vi "RT.vi"() -> ()   [LabVIEW 2015]
uses:
  <vilib>/FPGAPlugInAG/sbRIO-9637/niLvFpga_Open_sbRIO-9637.vi
  <vilib>/rvi/interface/common/dynamic/niFpgaDynamicAddResources.vi
  <vilib>/Utility/error.llb/Error Cluster From Error Code.vi
  <vilib>/rvi/errors/niLvFpgaAdjustHostInterfaceError.vi
  <vilib>/FPGAPlugInAG/Dynamic/niLvFpga_Close_Dynamic.vi
  <vilib>/EmbeddedDisplay/Hitachi HD44780/Host/Public/Output (String).vi
  <vilib>/rvi/interface/nirviOpenFPGA/nirviOpenFPGA.xnode
  FPGA Bitfiles/ECM-Project_FPGATarget_FPGA_qZxlCAm-DOY.lvbitx
  FPGA/FPGA.vi
  <vilib>/rvi/interface/nirviReadWriteControl/nirviReadWriteControl.xnode
  <vilib>/rvi/interface/nirviCloseFPGA/nirviCloseFPGA.xnode
  <vilib>/rvi/interface/nirviMethod/nirviMethod.xnode
  <vilib>/EmbeddedDisplay/Hitachi HD44780/Host/HD44780 Host.lvlib
  <vilib>/FPGAPlugInAG/Dynamic/niLvFpga_ReadFifo_Dynamic.vi
  <vilib>/rvi/errors/niLvFpgaMergeErrorWithErrorCode.vi
  NiFpgaLv.dll
  <vilib>/rvi/interface/Simulation/niFpgaSimulationCallBeginRW.vi
panel:
  out "Gauge":dbl(knob) scale=0.0..10.0
  out "Meter":dbl(knob) scale=0.0..5.0
  in  "Port":u16=2055 min=1025 step=1
  in  "Clear LCD":bool
  in  "Slide":dbl(slide) scale=0.0..10.0
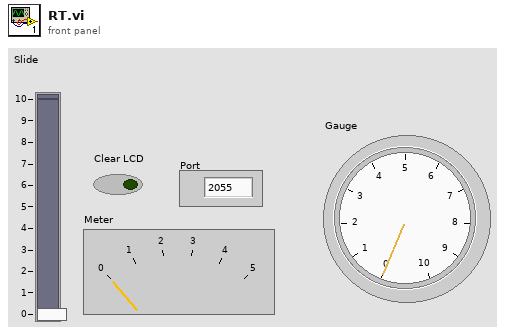
[diagram p1: front panel]
types:
  T1 = enum8{"5x8 & 2 lines", "5x10 & 1 line", "5x8 & 1 line"}
  T2 = enum8{"8x1", "8x2", "12x4", "16x1", "16x2", "16x4", "20x1", "20x2", "20x4", "24x1", "24x2", "40x2", "40x4"}
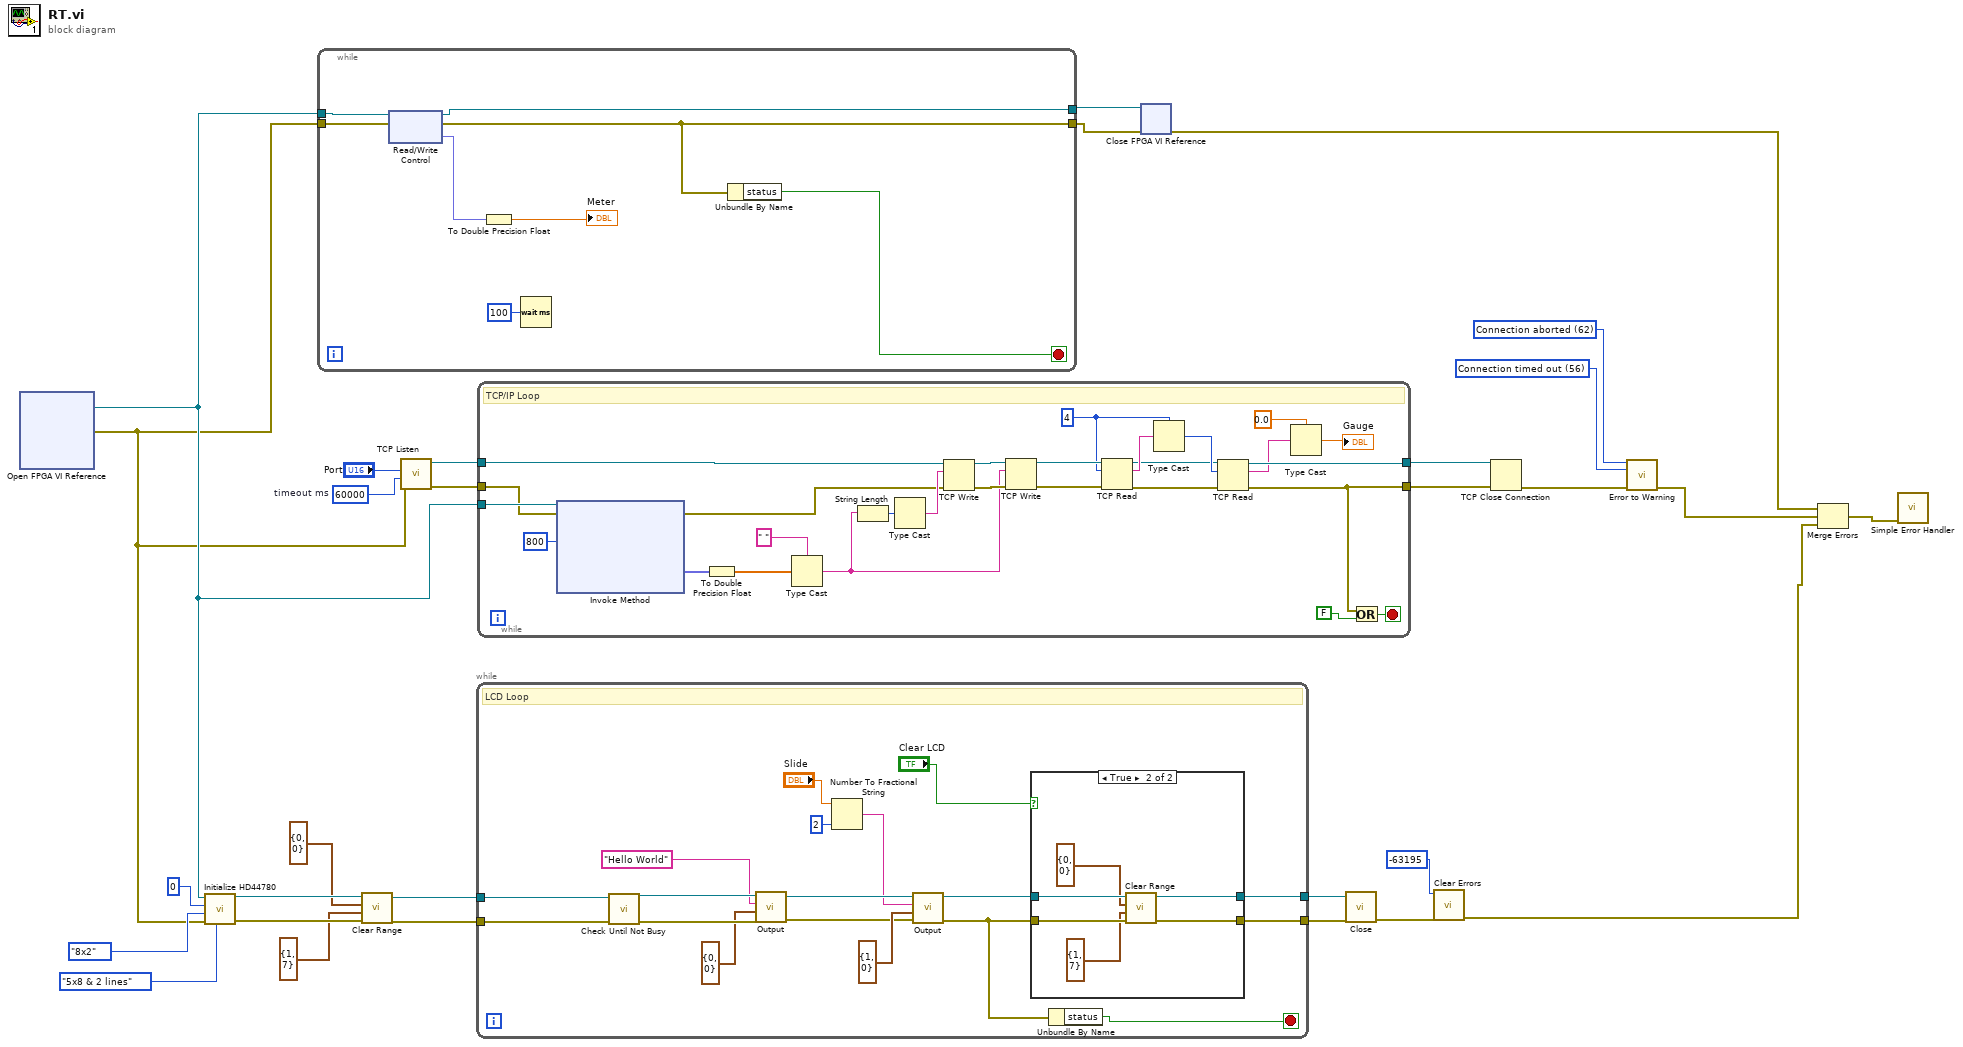
[diagram p0: block diagram]
diagram:
  w17 = 60000  # timeout ms
  w12 = 56 items=["No Error", "Argument Error", "Memory Full", "Out of Zone", "End of File", "File Already Open", "Generic File IO Error", "File Not Found", "File Permission Error", "Disk Full", "Duplicate Path", "Too Many Files Open", "Not Enabled", "Resource File Not Found", "Cannot Add Resource", "Resource Not Found", "Image Not Found", "Image Memory Error", "Pen Does Not Exist", "Config Bad Type", "Config Token Not Found", "Config Parse Error", "Config Memory Error", "Bad External Code Format", "Bad External Code Offset", "External Code Not Present", "Null Window", "Destroy Window Mixup", "Null Menu", "Print Aborted", "Bad Print Record", "Print Driver Error", "Windows Error During Print", "Memory Error During Print", "Print Dialog Error", "Generic Print Error", "Invalid Device Refnum", "Device Not Found", "Device Parameter Error", "Device Unit Error", "Can't Open Device", "Device Call Aborted", "Generic Error", "Cancelled By User", "Object ID Too Low", "Object ID Too High", "Object Not In Heap", "Unknown Heap", "Bad DefProc ID", "DefProc Not In Table", "Message Out Of Range", "Null Method", "Unknown Message", "Manager Call Not Supported", "Bad address", "Connection In progress", "Connection timed out", "Connection is already in progress", "Network attribute not supported", "Network error", "Address in use", "System out of memory", "Connection aborted", "Connection refused", "Connection is not connected", "Connection is already connected", "Connection closed", "Initialize error (interapplication manager)", "Bad occurrence", "Wait on unbound occurrence handler", "Occurrence queue overflow", "Bad path", "Semaphore not signaled", "Unrecognized type (interapplication manager)"] ("2nd Error to Convert")
  w11 = 62 items=["No Error", "Argument Error", "Memory Full", "Out of Zone", "End of File", "File Already Open", "Generic File IO Error", "File Not Found", "File Permission Error", "Disk Full", "Duplicate Path", "Too Many Files Open", "Not Enabled", "Resource File Not Found", "Cannot Add Resource", "Resource Not Found", "Image Not Found", "Image Memory Error", "Pen Does Not Exist", "Config Bad Type", "Config Token Not Found", "Config Parse Error", "Config Memory Error", "Bad External Code Format", "Bad External Code Offset", "External Code Not Present", "Null Window", "Destroy Window Mixup", "Null Menu", "Print Aborted", "Bad Print Record", "Print Driver Error", "Windows Error During Print", "Memory Error During Print", "Print Dialog Error", "Generic Print Error", "Invalid Device Refnum", "Device Not Found", "Device Parameter Error", "Device Unit Error", "Can't Open Device", "Device Call Aborted", "Generic Error", "Cancelled By User", "Object ID Too Low", "Object ID Too High", "Object Not In Heap", "Unknown Heap", "Bad DefProc ID", "DefProc Not In Table", "Message Out Of Range", "Null Method", "Unknown Message", "Manager Call Not Supported", "Bad address", "Connection In progress", "Connection timed out", "Connection is already in progress", "Network attribute not supported", "Network error", "Address in use", "System out of memory", "Connection aborted", "Connection refused", "Connection is not connected", "Connection is already connected", "Connection closed", "Initialize error (interapplication manager)", "Bad occurrence", "Wait on unbound occurrence handler", "Occurrence queue overflow", "Bad path", "Semaphore not signaled", "Unrecognized type (interapplication manager)"] ("1st Error to Convert")
  n1 = xnode "Open FPGA VI Reference"() -> ("FPGA VI Reference Out"=w5:refnum<k20>, "error out"=w4:errorcluster)  [unwired: 2 in]
  n2 = call <vilib>:"Initialize HD44780.vi"("font configuration (5x8 & 2 lines)"=T1."5x8 & 2 lines", "error in (no error)"=w4, "screen size"=T2."8x2", "device index"=i8 0, "FPGA VI Reference in"=w5) -> ("error out"=w21:errorcluster, "LCD out"=w20:refnum<class "Character LCD.lvclass">)  [unwired: 5 in]
  n3 = while {
    tunnel: w5 -> [w38]
    tunnel: w4 -> [w37]
    tunnel: [w33] -> w3
    tunnel: [w32] -> w2
    stop <- w34 stop-if-true
    n4 = xnode "Read/Write Control"("FPGA VI Reference In"=w38, "error in"=w37) -> ("FPGA VI Reference Out"=w33:refnum<k20>, "error out"=w32:errorcluster, "POT"=w36:fxp<+/-,24,5>)
    n5 = To Double Precision Float(number=w36) -> (double precision float=→"Meter":dbl)
    n6 = Wait (ms)(milliseconds to wait=u32 100) -> ()  [unwired: 1 out]
    n7 = Unbundle By Name(w32) -> ("status"=w34:bool)
  }
  n8 = call <vilib>:"Clear Range.vi"("error in (no error)"=w21, "end position (end of line)"=cluster{"row":i8, "column":i8} {"row"=1, "column"=7}, "start position"=cluster{"row":i8, "column":i8} {"row"=0, "column"=0}, "LCD in"=w20) -> ("error out"=w23:errorcluster, "LCD out"=w22:refnum<class "Character LCD.lvclass">)  [unwired: 6 in]
  n9 = call <vilib>:"TCP Listen.vi"("error in (no error)"=w4, "timeout ms (wait forever: -1)"=w17, "port"="Port") -> ("error out"=w16:errorcluster, "connection ID"=w14:refnum<k5>)  [unwired: 1 in, 6 out]
  n10 = while {
    tunnel: w22 -> [w55]
    tunnel: w23 -> [w56]
    tunnel: [w42] -> w25
    tunnel: [w41] -> w24
    stop <- w39 stop-if-true
    # "LCD Loop"
    n11 = call "Check Until Not Busy.vi"("error in"=w56, "LCD in"=w55) -> ("error out"=w54:errorcluster, "LCD out"=w53:refnum<class "Character LCD.lvclass">)  [unwired: 8 in]
    n12 = call-poly <vilib>:"Output.vi"("error in (no error)"=w54, "position"=cluster{"row":i8, "column":i8} {"row"=0, "column"=0}, "text"="Hello World" ("String"), "LCD in"=w53) -> ("error out"=w50:errorcluster, "LCD out"=w49:refnum<class "Character LCD.lvclass">)  [unwired: 5 in, 1 out]
    n13 = Number To Fractional String(number="Slide", precision (6)=i16 2) -> (F-format string=w46:string)  [unwired: 2 in]
    n14 = call-poly <vilib>:"Output.vi"("error in (no error)"=w50, "position"=cluster{"row":i8, "column":i8} {"row"=1, "column"=0}, "text"=w46, "LCD in"=w49) -> ("error out"=w40:errorcluster, "LCD out"=w43:refnum<class "Character LCD.lvclass">)  [unwired: 5 in, 1 out]
    n15 = case shown="True" "Clear LCD" {
      tunnel: w43 -> [w58 w64]
      tunnel: w40 -> [w57 w63]
      tunnel: [w57 w62] -> w42
      tunnel: [w58 w61] -> w41
      frame False {
      }
      frame True {
        n16 = call <vilib>:"Clear Range.vi"("error in (no error)"=w63, "end position (end of line)"=cluster{"row":i8, "column":i8} {"row"=1, "column"=7}, "start position"=cluster{"row":i8, "column":i8} {"row"=0, "column"=0}, "LCD in"=w64) -> ("error out"=w62:errorcluster, "LCD out"=w61:refnum<class "Character LCD.lvclass">)  [unwired: 6 in]
      }
    }
    n17 = Unbundle By Name(w40) -> ("status"=w39:bool)
  }
  n18 = while {
    tunnel: [w74] -> w15
    tunnel: [w73] -> w13
    tunnel: w14 -> [w91]
    tunnel: w16 -> [w82]
    tunnel: w5 -> [w83]
    stop <- w85 stop-if-true
    w70 = 4
    # "TCP/IP Loop"
    n19 = xnode "Invoke Method"("FPGA VI Reference In"=w83, "error in"=w82, "Number of Elements"=u32 800) -> ("error out"=w81:errorcluster, "Data"=w78:fxp<+/-,24,5>[])  [unwired: 1 in, 2 out]
    n20 = To Double Precision Float(number=w78) -> (double precision float=w77:dbl[])
    n21 = Type Cast(type=" ", x=w77) -> (*(type *) &x=w86:string)
    n22 = String Length(string=w86) -> (length=w88:i32)
    n23 = Type Cast(x=w88) -> (*(type *) &x=w87:string)  [unwired: 1 out]
    n24 = TCP Write(connection ID=w91, data in=w87, error in (no error)=w81) -> (connection ID out=w90:refnum<k5>, error out=w89:errorcluster)  [unwired: 2 out]
    n25 = TCP Write(connection ID=w90, data in=w86, error in (no error)=w89) -> (connection ID out=w75:refnum<k5>, error out=w76:errorcluster)  [unwired: 2 out]
    n26 = TCP Read(connection ID=w75, bytes to read=w70, error in (no error)=w76) -> (connection ID out=w69:refnum<k5>, data out=w72:string, error out=w68:errorcluster)  [unwired: 2 in]
    n27 = Type Cast(type=w70, x=w72) -> (*(type *) &x=w71:i32)
    n28 = TCP Read(connection ID=w69, bytes to read=w71, error in (no error)=w68) -> (connection ID out=w73:refnum<k5>, data out=w65:string, error out=w74:errorcluster)  [unwired: 2 in]
    n29 = Type Cast(type=0.0, x=w65) -> (*(type *) &x=→"Gauge":dbl)
    n30 = Or(x=w74, y=FALSE) -> (x .or. y?=w85:bool)
  }
  n31 = xnode "Close FPGA VI Reference"("FPGA VI Reference In"=w3, "error in"=w2) -> ("error out"=w1:errorcluster)
  n32 = call <vilib>:"Close.vi"("error in (no error)"=w25, "LCD in"=w24) -> ("error out"=w27:errorcluster)  [unwired: 9 in]
  n33 = call <vilib>:"Clear Errors.vi"("error in (no error)"=w27, "specific error code to clear (0: all)"=-63195) -> ("error out"=w7:errorcluster)  [unwired: 4 in, 1 out]
  n34 = TCP Close Connection(connection ID=w13, error in (no error)=w15) -> (error out=w10:errorcluster)  [unwired: 2 out]
  n35 = call <vilib>:"Error to Warning.vi"("1st Error to Convert"=w11, "2nd Error to Convert"=w12, "error in"=w10) -> ("warning out"=w6:errorcluster)  [unwired: 3 in, 9 out]
  n36 = Merge Errors(w1, w6, w7) -> (w8:errorcluster)
  n37 = call <vilib>:"Simple Error Handler.vi"("error in (no error)"=w8) -> ()  [unwired: 1 in, 8 out]
